vi "MB Ethernet Check Client.vi"(8 "error in (no error)":errorcluster, 10 "Remote Address":string, 11 "Connection ID in":refnum<k5>) -> (0 "error out":errorcluster, 2 "Priority":bool, 3 "Connection ID out":refnum<k5>)   [LabVIEW 2020]
uses:
  MB Globals.vi
panel:
  # "VI Name: MB Ethernet Check Client.vi\nPurpose: Verifies that the client trying to connect is allowed to connect to the server."
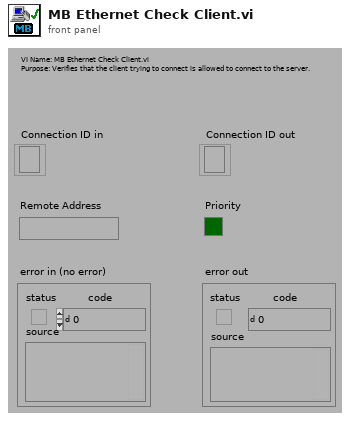
[diagram p1: front panel]
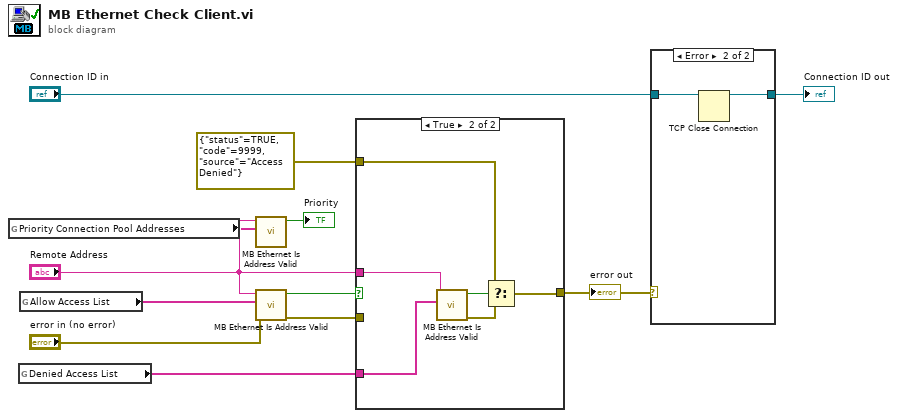
[diagram p0: block diagram]
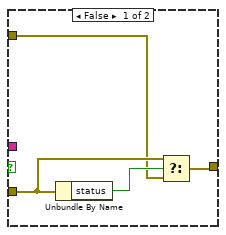
[diagram p2: hidden frame]
diagram:
  n1 = global read "MB Globals.vi" "Priority Connection Pool Addresses"() -> (w7:string[])
  n2 = global read "MB Globals.vi" "Denied Access List"() -> (w9:string[])
  n3 = global read "MB Globals.vi" "Allow Access List"() -> (w10:string[])
  n4 = call "MB Ethernet Is Address Valid.vi"("Valid IP Addresses"=w7, "IP Address"="Remote Address") -> ("IP Valid"=→"Priority":bool)  [unwired: 2 in, 7 out]
  n5 = call "MB Ethernet Is Address Valid.vi"("error in (no error)"="error in (no error)", "Valid IP Addresses"=w10, "IP Address"="Remote Address") -> ("error out"=w3:errorcluster, "IP Valid"=w4:bool)  [unwired: 1 in, 6 out]
  n6 = case shown="True" w4 {
    tunnel: "Remote Address" -> [_ w22]
    tunnel: w9 -> [_ w21]
    tunnel: [w13 w18] -> w1
    tunnel: w3 -> [w15 _]
    tunnel: errorcluster {"status"=TRUE, "code"=9999, "source"="Access Denied"} ("error out") -> [w14 w17]
    frame False {
      n7 = Unbundle By Name(w15) -> ("status"=w16:bool)
      n8 = Select(t=w15, s=w16, f=w14) -> (s? t:f=w13:errorcluster)
    }
    frame True {
      n9 = call "MB Ethernet Is Address Valid.vi"("Valid IP Addresses"=w21, "IP Address"=w22) -> ("error out"=w19:errorcluster, "IP Valid"=w20:bool)  [unwired: 1 in, 7 out]
      n10 = Select(t=w17, s=w20, f=w19) -> (s? t:f=w18:errorcluster)
    }
  }
  "error out" <- w1
  n11 = case shown="Error" w1 {
    tunnel: "Connection ID in" -> [w23 w25]
    tunnel: [w23 w24] -> w11
    frame No Error {
    }
    frame Error {
      n12 = TCP Close Connection(connection ID=w25) -> (connection ID out=w24:refnum<k5>)  [unwired: 1 in, 2 out]
    }
  }
  "Connection ID out" <- w11
